vi "Unit Conversion.vi"(5 "입력값 (옵션)":dbl, 7 "반올림 옵션":enum16{"없음", "반올림", "올림", "내림"}(ring), 8 "소수점 자리수":i32=-1, 9 "환산단위":string, 10 "입력단위":string, 11 "입력값":string) -> (0 "입력단위":string, 1 "환산단위":string, 2 "환산값 (DBL)":dbl format="%#.6f", 3 "환산값 (string)":string, 4 "환산단위 오류":bool, 6 "입력단위 오류":bool)   [LabVIEW 2020]
uses:
  Variables/Global_Constant.vi
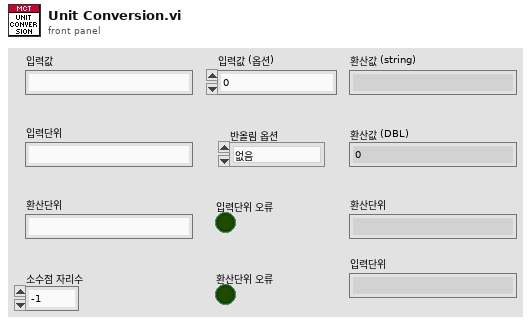
[diagram p1: front panel]
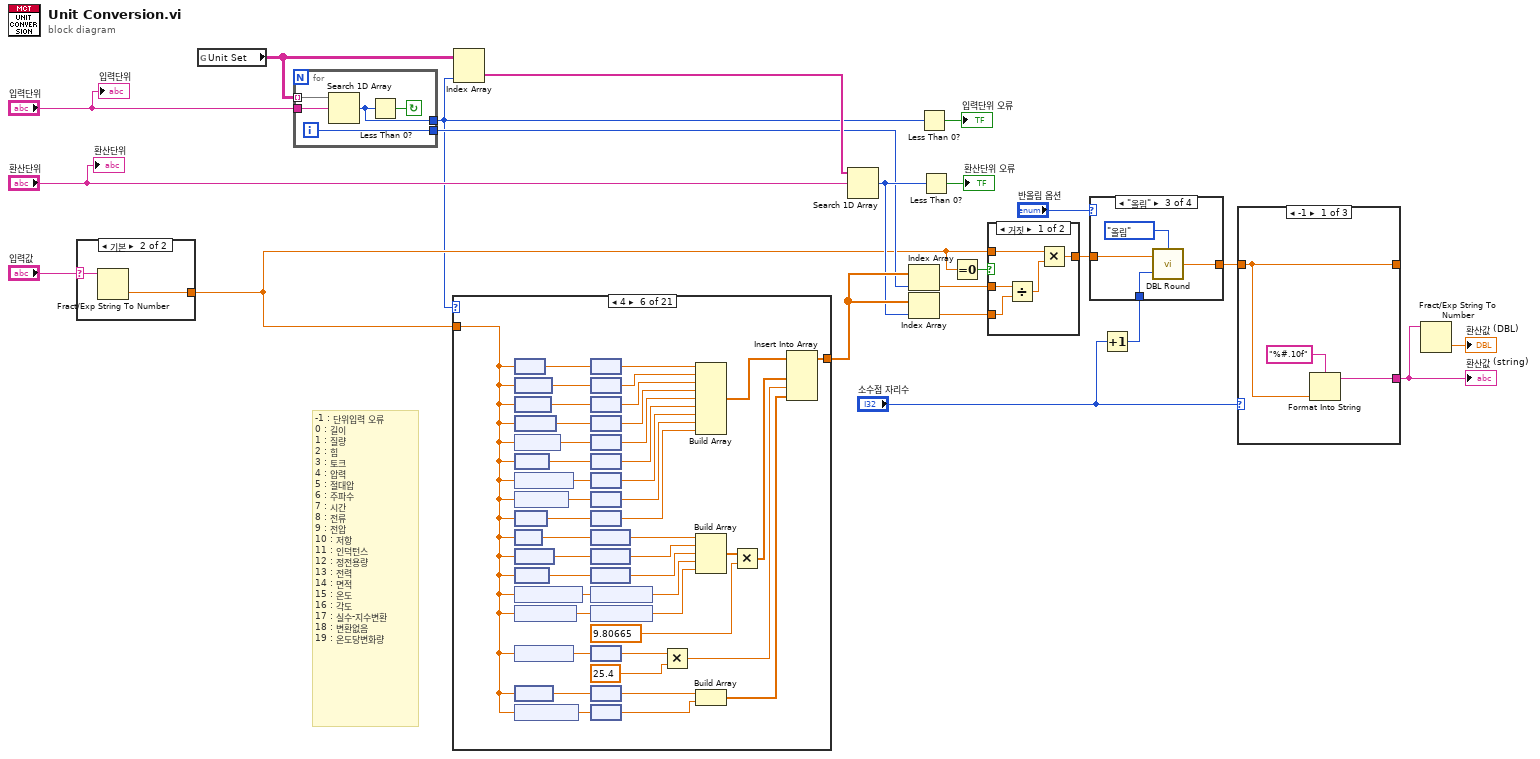
[diagram p0: block diagram]
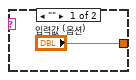
[diagram p2: hidden frame]
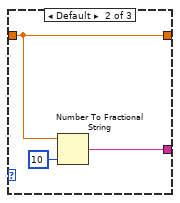
[diagram p4: hidden frame]
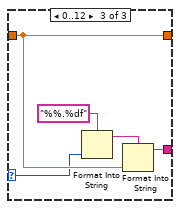
[diagram p5: hidden frame]
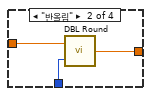
[diagram p7: hidden frame]
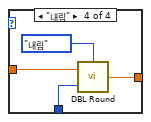
[diagram p8: hidden frame]
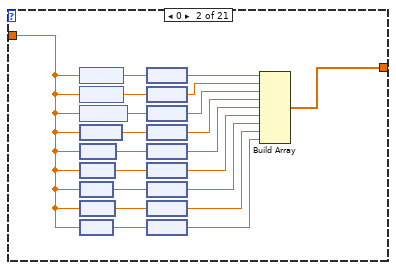
[diagram p10: hidden frame]
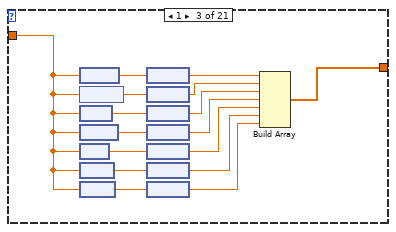
[diagram p11: hidden frame]
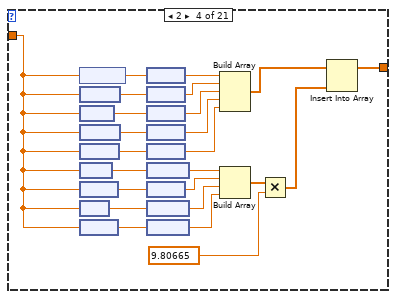
[diagram p12: hidden frame]
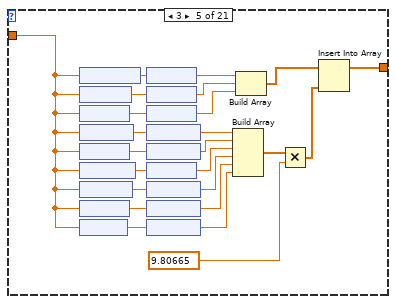
[diagram p13: hidden frame]
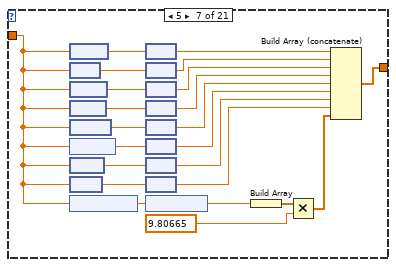
[diagram p14: hidden frame]
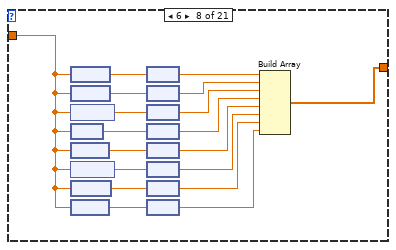
[diagram p15: hidden frame]
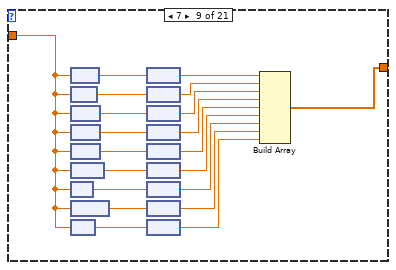
[diagram p16: hidden frame]
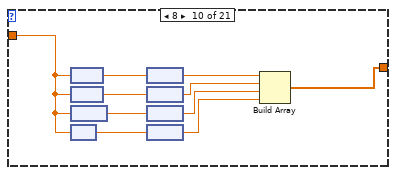
[diagram p17: hidden frame]
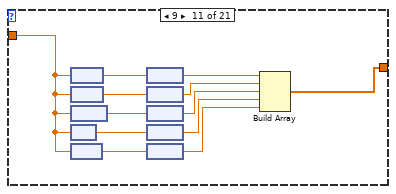
[diagram p18: hidden frame]
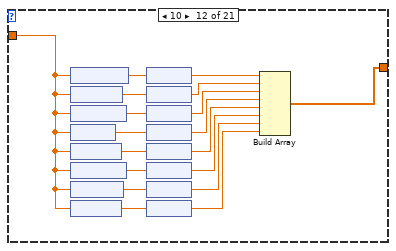
[diagram p19: hidden frame]
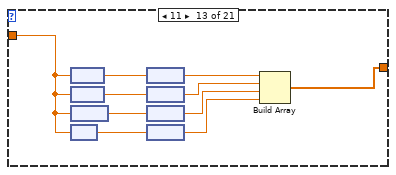
[diagram p20: hidden frame]
diagram:
  # "-1 : 단위입력 오류\n0 : 길이\n1 : 질량\n2 : 힘\n3 : 토크\n4 : 압력\n5 : 절대압\n6 : 주파수\n7 : 시간\n8 : 전류\n9 : 전압\n10 : 저항\n11 : 인덕턴스\n12 : 정전용량 \n13 : 전력\n14 : 면적\n15 : 온도\n16 : 각도\n17 : 실수-지수변환\n18 : 변환없음\n19 : 온도당변화량"
  n1 = case shown="기본" "입력값" {
    selector: "입력값" -> [_ w24]
    tunnel: ["입력값 (옵션)" w25] -> w10
    frame "" {
    }
    frame Default {
      n2 = Fract/Exp String To Number(string=w24) -> (number=w25:dbl)  [unwired: 3 in, 1 out]
    }
  }
  n3 = global read "Global_Constant.vi" "Unit Set"() -> (w6:string[][])
  n4 = for {
    tunnel: w6 -> [w30] mode=indexing
    tunnel: "입력단위" -> [w29]
    tunnel: [w27] -> w8
    tunnel: [w26] -> w12
    i -> [w26]
    stop <- w28 continue-if-true
    n5 = Search 1D Array(1D array=w30, element=w29) -> (index of element=w27:i32)  [unwired: 1 in]
    n6 = Less Than 0?(x=w27) -> (x < 0?=w28:bool)
  }
  n7 = case shown="4" w8 {
    tunnel: w10 -> [_ w33 w55 w67 w92 w116 w159 w182 w203 w219 w230 w242 w259 w271 w285 w293 w301 w313 w331 w337 w339]
    tunnel: [_ w36 w59 w70 w95 w142 w166 w190 w210 w221 w233 w251 w261 w277 w286 w294 w302 w324 w332 w338 w344] -> w22
    frame Default {
    }
    frame 0 {
      n8 = node(w33) -> (w50:dbl[unit])
      n9 = node(w33) -> (w49:dbl[unit])
      n10 = node(w33) -> (w48:dbl[unit])
      n11 = node(w33) -> (w47:dbl[unit])
      n12 = node(w33) -> (w46:dbl[unit])
      n13 = node(w33) -> (w45:dbl[unit])
      n14 = node(w33) -> (w44:dbl[unit])
      n15 = node(w33) -> (w34:dbl[unit])
      n16 = node(w33) -> (w35:dbl[unit])
      n17 = node(w50) -> (w43:dbl)
      n18 = node(w49) -> (w42:dbl)
      n19 = node(w48) -> (w41:dbl)
      n20 = node(w47) -> (w40:dbl)
      n21 = node(w46) -> (w39:dbl)
      n22 = node(w45) -> (w38:dbl)
      n23 = node(w44) -> (w37:dbl)
      n24 = node(w34) -> (w32:dbl)
      n25 = node(w35) -> (w31:dbl)
      n26 = Build Array(w43, w42, w41, w40, w39, w38, w37, w32, w31) -> (w36:dbl[])
    }
    frame 1 {
      n27 = node(w55) -> (w66:dbl[unit])
      n28 = node(w55) -> (w65:dbl[unit])
      n29 = node(w55) -> (w64:dbl[unit])
      n30 = node(w55) -> (w58:dbl[unit])
      n31 = node(w55) -> (w56:dbl[unit])
      n32 = node(w55) -> (w54:dbl[unit])
      n33 = node(w55) -> (w53:dbl[unit])
      n34 = node(w66) -> (w63:dbl)
      n35 = node(w65) -> (w62:dbl)
      n36 = node(w64) -> (w61:dbl)
      n37 = node(w58) -> (w60:dbl)
      n38 = node(w56) -> (w57:dbl)
      n39 = node(w54) -> (w52:dbl)
      n40 = node(w53) -> (w51:dbl)
      n41 = Build Array(w63, w62, w61, w60, w57, w52, w51) -> (w59:dbl[])
    }
    frame 2 {
      n42 = node(w67) -> (w90:dbl[unit])
      n43 = node(w67) -> (w69:dbl[unit])
      n44 = node(w67) -> (w89:dbl[unit])
      n45 = node(w67) -> (w88:dbl[unit])
      n46 = node(w67) -> (w87:dbl[unit])
      n47 = node(w67) -> (w85:dbl[unit])
      n48 = node(w67) -> (w82:dbl[unit])
      n49 = node(w67) -> (w84:dbl[unit])
      n50 = node(w67) -> (w83:dbl[unit])
      n51 = node(w90) -> (w81:dbl)
      n52 = node(w69) -> (w68:dbl)
      n53 = node(w89) -> (w80:dbl)
      n54 = node(w88) -> (w79:dbl)
      n55 = node(w87) -> (w86:dbl)
      n56 = node(w85) -> (w78:dbl)
      n57 = node(w82) -> (w77:dbl)
      n58 = node(w84) -> (w76:dbl)
      n59 = node(w83) -> (w75:dbl)
      n60 = Build Array(w81, w68, w80, w79, w86) -> (w72:dbl[])
      n61 = Build Array(w78, w77, w76, w75) -> (w74:dbl[])
      n62 = Multiply(x=w74, y=9.80665) -> (x*y=w71:dbl[])
      n63 = Insert Into Array(array=w72, new element=w71) -> (w70:dbl[])  [unwired: 1 in]
    }
    frame 3 {
      n64 = node(w92) -> (w114:dbl[unit])
      n65 = node(w92) -> (w113:dbl[unit])
      n66 = node(w92) -> (w112:dbl[unit])
      n67 = node(w92) -> (w111:dbl[unit])
      n68 = node(w92) -> (w110:dbl[unit])
      n69 = node(w92) -> (w107:dbl[unit])
      n70 = node(w92) -> (w109:dbl[unit])
      n71 = node(w92) -> (w108:dbl[unit])
      n72 = node(w92) -> (w93:dbl[unit])
      n73 = node(w114) -> (w106:dbl)
      n74 = node(w113) -> (w105:dbl)
      n75 = node(w112) -> (w104:dbl)
      n76 = node(w111) -> (w94:dbl)
      n77 = node(w110) -> (w103:dbl)
      n78 = node(w107) -> (w102:dbl)
      n79 = node(w109) -> (w101:dbl)
      n80 = node(w108) -> (w100:dbl)
      n81 = node(w93) -> (w91:dbl)
      n82 = Build Array(w94, w103, w102, w101, w100, w91) -> (w99:dbl[])
      n83 = Build Array(w106, w105, w104) -> (w97:dbl[])
      n84 = Multiply(x=w99, y=9.80665) -> (x*y=w96:dbl[])
      n85 = Insert Into Array(array=w97, new element=w96) -> (w95:dbl[])  [unwired: 1 in]
    }
    frame 4 {
      n86 = node(w116) -> (w157:dbl[unit])
      n87 = node(w116) -> (w156:dbl[unit])
      n88 = node(w116) -> (w155:dbl[unit])
      n89 = node(w116) -> (w154:dbl[unit])
      n90 = node(w116) -> (w153:dbl[unit])
      n91 = node(w116) -> (w150:dbl[unit])
      n92 = node(w116) -> (w152:dbl[unit])
      n93 = node(w116) -> (w151:dbl[unit])
      n94 = node(w116) -> (w141:dbl[unit])
      n95 = node(w116) -> (w126:dbl[unit])
      n96 = node(w116) -> (w135:dbl[unit])
      n97 = node(w116) -> (w132:dbl[unit])
      n98 = node(w116) -> (w130:dbl[unit])
      n99 = node(w116) -> (w128:dbl[unit])
      n100 = node(w116) -> (w124:dbl[unit])
      n101 = node(w116) -> (w120:dbl[unit])
      n102 = node(w116) -> (w117:dbl[unit])
      n103 = node(w157) -> (w149:dbl)
      n104 = node(w156) -> (w148:dbl)
      n105 = node(w155) -> (w147:dbl)
      n106 = node(w154) -> (w140:dbl)
      n107 = node(w153) -> (w139:dbl)
      n108 = node(w150) -> (w138:dbl)
      n109 = node(w152) -> (w137:dbl)
      n110 = node(w151) -> (w136:dbl)
      n111 = node(w141) -> (w134:dbl)
      n112 = node(w126) -> (w125:dbl)
      n113 = node(w135) -> (w133:dbl)
      n114 = node(w132) -> (w131:dbl)
      n115 = node(w130) -> (w129:dbl)
      n116 = node(w128) -> (w127:dbl)
      n117 = node(w124) -> (w123:dbl)
      n118 = node(w120) -> (w119:dbl)
      n119 = node(w117) -> (w115:dbl)
      n120 = Multiply(x=w123, y=25.4) -> (x*y=w122:dbl)
      n121 = Build Array(w149, w148, w147, w140, w139, w138, w137, w136, w134) -> (w144:dbl[])
      n122 = Build Array(w125, w133, w131, w129, w127) -> (w146:dbl[])
      n123 = Build Array(w119, w115) -> (w118:dbl[])
      n124 = Multiply(x=w146, y=9.80665) -> (x*y=w143:dbl[])
      n125 = Insert Into Array(array=w144, new element #1=w143, new element #2=w122, new element #3=w118) -> (w142:dbl[])  [unwired: 1 in]
    }
    frame 5 {
      n126 = node(w159) -> (w165:dbl[unit])
      n127 = node(w159) -> (w174:dbl[unit])
      n128 = node(w159) -> (w175:dbl[unit])
      n129 = node(w159) -> (w176:dbl[unit])
      n130 = node(w159) -> (w177:dbl[unit])
      n131 = node(w159) -> (w178:dbl[unit])
      n132 = node(w159) -> (w179:dbl[unit])
      n133 = node(w159) -> (w180:dbl[unit])
      n134 = node(w159) -> (w161:dbl[unit])
      n135 = node(w165) -> (w164:dbl)
      n136 = node(w174) -> (w173:dbl)
      n137 = node(w175) -> (w172:dbl)
      n138 = node(w176) -> (w171:dbl)
      n139 = node(w177) -> (w170:dbl)
      n140 = node(w178) -> (w169:dbl)
      n141 = node(w179) -> (w168:dbl)
      n142 = node(w180) -> (w167:dbl)
      n143 = node(w161) -> (w160:dbl)
      n144 = Build Array(w160) -> (w163:dbl[])
      n145 = Multiply(x=w163, y=9.80665) -> (x*y=w158:dbl[])
      n146 = Build Array (concatenate)(w164, w173, w172, w171, w170, w169, w168, w167, w158) -> (w166:dbl[])
    }
    frame 6 {
      n147 = node(w182) -> (w186:dbl[unit])
      n148 = node(w182) -> (w187:dbl[unit])
      n149 = node(w182) -> (w198:dbl[unit])
      n150 = node(w182) -> (w197:dbl[unit])
      n151 = node(w182) -> (w196:dbl[unit])
      n152 = node(w182) -> (w195:dbl[unit])
      n153 = node(w182) -> (w194:dbl[unit])
      n154 = node(w182) -> (w183:dbl[unit])
      n155 = node(w186) -> (w185:dbl)
      n156 = node(w187) -> (w184:dbl)
      n157 = node(w198) -> (w193:dbl)
      n158 = node(w197) -> (w192:dbl)
      n159 = node(w196) -> (w191:dbl)
      n160 = node(w195) -> (w189:dbl)
      n161 = node(w194) -> (w188:dbl)
      n162 = node(w183) -> (w181:dbl)
      n163 = Build Array(w185, w184, w193, w192, w191, w189, w188, w181) -> (w190:dbl[])
    }
    frame 7 {
      n164 = node(w203) -> (w218:dbl[unit])
      n165 = node(w203) -> (w217:dbl[unit])
      n166 = node(w203) -> (w216:dbl[unit])
      n167 = node(w203) -> (w215:dbl[unit])
      n168 = node(w203) -> (w214:dbl[unit])
      n169 = node(w203) -> (w207:dbl[unit])
      n170 = node(w203) -> (w206:dbl[unit])
      n171 = node(w203) -> (w205:dbl[unit])
      n172 = node(w203) -> (w204:dbl[unit])
      n173 = node(w218) -> (w213:dbl)
      n174 = node(w217) -> (w212:dbl)
      n175 = node(w216) -> (w211:dbl)
      n176 = node(w215) -> (w209:dbl)
      n177 = node(w214) -> (w208:dbl)
      n178 = node(w207) -> (w202:dbl)
      n179 = node(w206) -> (w201:dbl)
      n180 = node(w205) -> (w200:dbl)
      n181 = node(w204) -> (w199:dbl)
      n182 = Build Array(w213, w212, w211, w209, w208, w202, w201, w200, w199) -> (w210:dbl[])
    }
    frame 8 {
      n183 = node(w219) -> (w228:dbl[unit])
      n184 = node(w219) -> (w227:dbl[unit])
      n185 = node(w219) -> (w226:dbl[unit])
      n186 = node(w219) -> (w225:dbl[unit])
      n187 = node(w228) -> (w224:dbl)
      n188 = node(w227) -> (w223:dbl)
      n189 = node(w226) -> (w222:dbl)
      n190 = node(w225) -> (w220:dbl)
      n191 = Build Array(w224, w223, w222, w220) -> (w221:dbl[])
    }
    frame 9 {
      n192 = node(w230) -> (w240:dbl[unit])
      n193 = node(w230) -> (w239:dbl[unit])
      n194 = node(w230) -> (w238:dbl[unit])
      n195 = node(w230) -> (w237:dbl[unit])
      n196 = node(w230) -> (w231:dbl[unit])
      n197 = node(w240) -> (w236:dbl)
      n198 = node(w239) -> (w235:dbl)
      n199 = node(w238) -> (w234:dbl)
      n200 = node(w237) -> (w232:dbl)
      n201 = node(w231) -> (w229:dbl)
      n202 = Build Array(w236, w235, w234, w232, w229) -> (w233:dbl[])
    }
    frame 10 {
      n203 = node(w242) -> (w258:dbl[unit])
      n204 = node(w242) -> (w257:dbl[unit])
      n205 = node(w242) -> (w256:dbl[unit])
      n206 = node(w242) -> (w255:dbl[unit])
      n207 = node(w242) -> (w249:dbl[unit])
      n208 = node(w242) -> (w247:dbl[unit])
      n209 = node(w242) -> (w245:dbl[unit])
      n210 = node(w242) -> (w243:dbl[unit])
      n211 = node(w258) -> (w254:dbl)
      n212 = node(w257) -> (w253:dbl)
      n213 = node(w256) -> (w252:dbl)
      n214 = node(w255) -> (w250:dbl)
      n215 = node(w249) -> (w248:dbl)
      n216 = node(w247) -> (w246:dbl)
      n217 = node(w245) -> (w244:dbl)
      n218 = node(w243) -> (w241:dbl)
      n219 = Build Array(w254, w253, w252, w250, w248, w246, w244, w241) -> (w251:dbl[])
    }
    frame 11 {
      n220 = node(w259) -> (w268:dbl[unit])
      n221 = node(w259) -> (w267:dbl[unit])
      n222 = node(w259) -> (w266:dbl[unit])
      n223 = node(w259) -> (w265:dbl[unit])
      n224 = node(w268) -> (w264:dbl)
      n225 = node(w267) -> (w263:dbl)
      n226 = node(w266) -> (w262:dbl)
      n227 = node(w265) -> (w260:dbl)
      n228 = Build Array(w264, w263, w262, w260) -> (w261:dbl[])
    }
    frame 12 {
      n229 = node(w271) -> (w284:dbl[unit])
      n230 = node(w271) -> (w283:dbl[unit])
      n231 = node(w271) -> (w282:dbl[unit])
      n232 = node(w271) -> (w281:dbl[unit])
      n233 = node(w271) -> (w275:dbl[unit])
      n234 = node(w271) -> (w273:dbl[unit])
      n235 = node(w271) -> (w272:dbl[unit])
      n236 = node(w284) -> (w280:dbl)
      n237 = node(w283) -> (w279:dbl)
      n238 = node(w282) -> (w278:dbl)
      n239 = node(w281) -> (w276:dbl)
      n240 = node(w275) -> (w274:dbl)
      n241 = node(w273) -> (w270:dbl)
      n242 = node(w272) -> (w269:dbl)
      n243 = Build Array(w280, w279, w278, w276, w274, w270, w269) -> (w277:dbl[])
    }
    frame 13 {
      n244 = node(w285) -> (w292:dbl[unit])
      n245 = node(w285) -> (w291:dbl[unit])
      n246 = node(w285) -> (w290:dbl[unit])
      n247 = node(w292) -> (w289:dbl)
      n248 = node(w291) -> (w288:dbl)
      n249 = node(w290) -> (w287:dbl)
      n250 = Build Array(w289, w288, w287) -> (w286:dbl[])
    }
    frame 14 {
      n251 = node(w293) -> (w300:dbl[unit])
      n252 = node(w293) -> (w299:dbl[unit])
      n253 = node(w293) -> (w298:dbl[unit])
      n254 = node(w300) -> (w297:dbl)
      n255 = node(w299) -> (w296:dbl)
      n256 = node(w298) -> (w295:dbl)
      n257 = Build Array(w297, w296, w295) -> (w294:dbl[])
    }
    frame 15 {
      n258 = node(w301) -> (w308:dbl[unit])
      n259 = node(w301) -> (w307:dbl[unit])
      n260 = node(w301) -> (w306:dbl[unit])
      n261 = node(w308) -> (w305:dbl)
      n262 = node(w307) -> (w304:dbl)
      n263 = node(w306) -> (w303:dbl)
      n264 = Build Array(w305, w304, w303) -> (w302:dbl[])
    }
    frame 16 {
      n265 = Divide(x=w313, y=1000.0) -> (x/y=w319:dbl)
      n266 = Divide(x=w313, y=1000000.0) -> (x/y=w316:dbl)
      n267 = Divide(x=w313, y=100.0) -> (x/y=w315:dbl)
      n268 = node(w313) -> (w330:dbl[unit])
      n269 = node(w313) -> (w329:dbl[unit])
      n270 = node(w313) -> (w328:dbl[unit])
      n271 = node(w313) -> (w323:dbl[unit])
      n272 = node(w319) -> (w320:dbl[unit])
      n273 = node(w316) -> (w318:dbl[unit])
      n274 = node(w315) -> (w317:dbl[unit])
      n275 = node(w330) -> (w327:dbl)
      n276 = node(w329) -> (w326:dbl)
      n277 = node(w328) -> (w325:dbl)
      n278 = node(w323) -> (w322:dbl)
      n279 = node(w320) -> (w311:dbl)
      n280 = node(w318) -> (w310:dbl)
      n281 = node(w317) -> (w309:dbl)
      n282 = Build Array(w327, w326, w325, w322, w311, w310, w309) -> (w324:dbl[])
    }
    frame 17 {
      n283 = node(w331) -> (w336:dbl[unit])
      n284 = node(w331) -> (w335:dbl[unit])
      n285 = node(w336) -> (w334:dbl)
      n286 = node(w335) -> (w333:dbl)
      n287 = Build Array(w331, w334, w333, w331) -> (w332:dbl[])
    }
    frame 18 {
      n288 = Build Array(w337, w337, w337, w337, w337, w337, w337, w337) -> (w338:dbl[])
    }
    frame 19 {
      n289 = Divide(x=w339, y=1000000.0) -> (x/y=w342:dbl)
      n290 = Divide(x=w339, y=100.0) -> (x/y=w340:dbl)
      n291 = Build Array(w342, w340, w339) -> (w344:dbl[])
    }
  }
  n292 = Index Array(array=w6, index (col)=w8) -> (element=w13:string[])  [unwired: 1 in]
  n293 = Search 1D Array(1D array=w13, element="환산단위") -> (index of element=w17:i32)  [unwired: 1 in]
  n294 = Index Array(array=w22, index=w12) -> (element=w14:dbl)
  n295 = Index Array(array=w22, index=w17) -> (element=w15:dbl)
  n296 = Less Than 0?(x=w8) -> (x < 0?=→"입력단위 오류":bool)
  n297 = Less Than 0?(x=w17) -> (x < 0?=→"환산단위 오류":bool)
  n298 = Equal To 0?(x=w10) -> (x = 0?=w9:bool)
  n299 = case shown="거짓" w9 {
    tunnel: [w349 w350] -> w20
    tunnel: w15 -> [w346 _]
    tunnel: w14 -> [w347 _]
    tunnel: w10 -> [w348 w350]
    frame False {
      n300 = Divide(x=w347, y=w346) -> (x/y=w345:dbl)
      n301 = Multiply(x=w348, y=w345) -> (x*y=w349:dbl)
    }
    frame True {
    }
  }
  n302 = Increment(x="소수점 자리수") -> (x+1=w4:i32)
  n303 = case shown="\"올림\"" "반올림 옵션" {
    tunnel: w20 -> [w351 w354 w358 w362]
    tunnel: [w351 w353 w357 w361] -> w11
    tunnel: w4 -> [_ w352 w356 w360]
    frame Default {
    }
    frame "반올림" {
      n304 = call "DBL Round.vi"("반올림자리수"=w352, "DBL in"=w354) -> ("DBL out"=w353:dbl)  [unwired: 1 in]
    }
    frame "올림" {
      n305 = call "DBL Round.vi"("반올림 옵션"=enum16{"반올림", "올림", "내림"}."올림", "반올림자리수"=w356, "DBL in"=w358) -> ("DBL out"=w357:dbl)
    }
    frame "내림" {
      n306 = call "DBL Round.vi"("반올림 옵션"=enum16{"반올림", "올림", "내림"}."내림", "반올림자리수"=w360, "DBL in"=w362) -> ("DBL out"=w361:dbl)
    }
  }
  n307 = case shown="-1" "소수점 자리수" {
    selector: "소수점 자리수" -> [_ _ w372]
    tunnel: [w364 w368 w369] -> w2
    tunnel: w11 -> [w363 w367 w373]
    tunnel: [w363 w367 w373] -> _
    frame -1 {
      n308 = Format Into String(format string="%#.10f" ("포맷 문자열"), w363) -> (resulting string=w364:string)  [unwired: 2 in, 1 out]
    }
    frame Default {
      n309 = Number To Fractional String(number=w367, precision (6)=i16 10 ("정밀도(6)")) -> (F-format string=w368:string)  [unwired: 2 in]
    }
    frame 0..12 {
      n310 = Format Into String(format string="%%.%df" ("포맷 문자열"), w372) -> (resulting string=w370:string)  [unwired: 2 in, 1 out]
      n311 = Format Into String(format string=w370, w373) -> (resulting string=w369:string)  [unwired: 2 in, 1 out]
    }
  }
  "환산값 (string)" <- w2
  n312 = Fract/Exp String To Number(string=w2) -> (number=→"환산값 (DBL)":dbl)  [unwired: 3 in, 1 out]
  "환산단위" <- "환산단위"
  "입력단위" <- "입력단위"
